vi "App - analyze RUS V6.vi"() -> ()   [LabVIEW 2021] (continued)
"Magn Field(T) "=0.0}, {"temperature"=14.72, "temperature str"="14.72000", "file path"=path "D:/Data/Ultrasound/LSCO/LSCO22__130814c/5_Cooling_2nd_try/September_2014/091714/14.72000K_500_2500_2.10000V_0.00000T_Sep17-2014__22-56-35_001_091714.bin", "last mod"=timestamp(3493853795 s since 1904-01-01), "file name str"="D:\\Data\\Ultrasound\\LSCO\\LSCO22__130814c\\5_Cooling_2nd_try\\September_2014\\091714\\14.72000K_500_2500_2.10000V_0.00000T_Sep17-2014__22-56-35_001_091714.bin", "mod time(min)"=58230896.583333336, "file format"=enum."binary", "power(V)"=2.1, "Magn Field(T) "=0.0}, {"temperature"=14.716, "temperature str"="14.71600", "file path"=path "D:/Data/Ultrasound/LSCO/LSCO22__130814c/5_Cooling_2nd_try/September_2014/091714/14.71600K_500_2500_2.10000V_0.00000T_Sep17-2014__22-57-54_001_091714.bin", "last mod"=timestamp(3493853874 s since 1904-01-01), "file name str"="D:\\Data\\Ultrasound\\LSCO\\LSCO22__130814c\\5_Cooling_2nd_try\\September_2014\\091714\\14.71600K_500_2500_2.10000V_0.00000T_Sep17-2014__22-57-54_001_091714.bin", "mod time(min)"=58230897.9, "file format"=enum."binary", "power(V)"=2.1, "Magn Field(T) "=0.0}, {"temperature"=14.713, "temperature str"="14.71300", "file path"=path "D:/Data/Ultrasound/LSCO/LSCO22__130814c/5_Cooling_2nd_try/September_2014/091714/14.71300K_500_2500_2.10000V_0.00000T_Sep17-2014__22-59-13_001_091714.bin", "last mod"=timestamp(3493853953 s since 1904-01-01), "file name str"="D:\\Data\\Ultrasound\\LSCO\\LSCO22__130814c\\5_Cooling_2nd_try\\September_2014\\091714\\14.71300K_500_2500_2.10000V_0.00000T_Sep17-2014__22-59-13_001_091714.bin", "mod time(min)"=58230899.21666667, "file format"=enum."binary", "power(V)"=2.1, "Magn Field(T) "=0.0}, {"temperature"=14.71, "temperature str"="14.71000", "file path"=path "D:/Data/Ultrasound/LSCO/LSCO22__130814c/5_Cooling_2nd_try/September_2014/091714/14.71000K_500_2500_2.10000V_0.00000T_Sep17-2014__23-00-33_001_091714.bin", "last mod"=timestamp(3493854033 s since 1904-01-01), "file name str"="D:\\Data\\Ultrasound\\LSCO\\LSCO22__130814c\\5_Cooling_2nd_try\\September_2014\\091714\\14.71000K_500_2500_2.10000V_0.00000T_Sep17-2014__23-00-33_001_091714.bin", "mod time(min)"=58230900.55, "file format"=enum."binary", "power(V)"=2.1, "Magn Field(T) "=0.0}, {"temperature"=14.704, "temperature str"="14.70400", "file path"=path "D:/Data/Ultrasound/LSCO/LSCO22__130814c/5_Cooling_2nd_try/September_2014/091714/14.70400K_500_2500_2.10000V_0.00000T_Sep17-2014__23-01-52_001_091714.bin", "last mod"=timestamp(3493854112 s since 1904-01-01), "file name str"="D:\\Data\\Ultrasound\\LSCO\\LSCO22__130814c\\5_Cooling_2nd_try\\September_2014\\091714\\14.70400K_500_2500_2.10000V_0.00000T_Sep17-2014__23-01-52_001_091714.bin", "mod time(min)"=58230901.86666667, "file format"=enum."binary", "power(V)"=2.1, "Magn Field(T) "=0.0}, {"temperature"=14.705, "temperature str"="14.70500", "file path"=path "D:/Data/Ultrasound/LSCO/LSCO22__130814c/5_Cooling_2nd_try/September_2014/091714/14.70500K_500_2500_2.10000V_0.00000T_Sep17-2014__23-03-11_001_091714.bin", "last mod"=timestamp(3493854191 s since 1904-01-01), "file name str"="D:\\Data\\Ultrasound\\LSCO\\LSCO22__130814c\\5_Cooling_2nd_try\\September_2014\\091714\\14.70500K_500_2500_2.10000V_0.00000T_Sep17-2014__23-03-11_001_091714.bin", "mod time(min)"=58230903.18333333, "file format"=enum."binary", "power(V)"=2.1, "Magn Field(T) "=0.0}, {"temperature"=14.703, "temperature str"="14.70300", "file path"=path "D:/Data/Ultrasound/LSCO/LSCO22__130814c/5_Cooling_2nd_try/September_2014/091714/14.70300K_500_2500_2.10000V_0.00000T_Sep17-2014__23-04-31_001_091714.bin", "last mod"=timestamp(3493854271 s since 1904-01-01), "file name str"="D:\\Data\\Ultrasound\\LSCO\\LSCO22__130814c\\5_Cooling_2nd_try\\September_2014\\091714\\14.70300K_500_2500_2.10000V_0.00000T_Sep17-2014__23-04-31_001_091714.bin", "mod time(min)"=58230904.516666666, "file format"=enum."binary", "power(V)"=2.1, "Magn Field(T) "=0.0}, {"temperature"=14.7, "temperature str"="14.70000", "file path"=path "D:/Data/Ultrasound/LSCO/LSCO22__130814c/5_Cooling_2nd_try/September_2014/091714/14.70000K_500_2500_2.10000V_0.00000T_Sep17-2014__23-05-50_001_091714.bin", "last mod"=timestamp(3493854350 s since 1904-01-01), "file name str"="D:\\Data\\Ultrasound\\LSCO\\LSCO22__130814c\\5_Cooling_2nd_try\\September_2014\\091714\\14.70000K_500_2500_2.10000V_0.00000T_Sep17-2014__23-05-50_001_091714.bin", "mod time(min)"=58230905.833333336, "file format"=enum."binary", "power(V)"=2.1, "Magn Field(T) "=0.0}, {"temperature"=14.697, "temperature str"="14.69700", "file path"=path "D:/Data/Ultrasound/LSCO/LSCO22__130814c/5_Cooling_2nd_try/September_2014/091714/14.69700K_500_2500_2.10000V_0.00000T_Sep17-2014__23-07-10_001_091714.bin", "last mod"=timestamp(3493854430 s since 1904-01-01), "file name str"="D:\\Data\\Ultrasound\\LSCO\\LSCO22__130814c\\5_Cooling_2nd_try\\September_2014\\091714\\14.69700K_500_2500_2.10000V_0.00000T_Sep17-2014__23-07-10_001_091714.bin", "mod time(min)"=58230907.166666664, "file format"=enum."binary", "power(V)"=2.1, "Magn Field(T) "=0.0}, {"temperature"=14.688, "temperature str"="14.68800", "file path"=path "D:/Data/Ultrasound/LSCO/LSCO22__130814c/5_Cooling_2nd_try/September_2014/091714/14.68800K_500_2500_2.10000V_0.00000T_Sep17-2014__23-08-29_001_091714.bin", "last mod"=timestamp(3493854509 s since 1904-01-01), "file name str"="D:\\Data\\Ultrasound\\LSCO\\LSCO22__130814c\\5_Cooling_2nd_try\\September_2014\\091714\\14.68800K_500_2500_2.10000V_0.00000T_Sep17-2014__23-08-29_001_091714.bin", "mod time(min)"=58230908.483333334, "file format"=enum."binary", "power(V)"=2.1, "Magn Field(T) "=0.0}, {"temperature"=14.695, "temperature str"="14.69500", "file path"=path "D:/Data/Ultrasound/LSCO/LSCO22__130814c/5_Cooling_2nd_try/September_2014/091714/14.69500K_500_2500_2.10000V_0.00000T_Sep17-2014__23-09-48_001_091714.bin", "last mod"=timestamp(3493854588 s since 1904-01-01), "file name str"="D:\\Data\\Ultrasound\\LSCO\\LSCO22__130814c\\5_Cooling_2nd_try\\September_2014\\091714\\14.69500K_500_2500_2.10000V_0.00000T_Sep17-2014__23-09-48_001_091714.bin", "mod time(min)"=58230909.8, "file format"=enum."binary", "power(V)"=2.1, "Magn Field(T) "=0.0}, {"temperature"=14.696, "temperature str"="14.69600", "file path"=path "D:/Data/Ultrasound/LSCO/LSCO22__130814c/5_Cooling_2nd_try/September_2014/091714/14.69600K_500_2500_2.10000V_0.00000T_Sep17-2014__23-11-08_001_091714.bin", "last mod"=timestamp(3493854668 s since 1904-01-01), "file name str"="D:\\Data\\Ultrasound\\LSCO\\LSCO22__130814c\\5_Cooling_2nd_try\\September_2014\\091714\\14.69600K_500_2500_2.10000V_0.00000T_Sep17-2014__23-11-08_001_091714.bin", "mod time(min)"=58230911.13333333, "file format"=enum."binary", "power(V)"=2.1, "Magn Field(T) "=0.0}, {"temperature"=14.691, "temperature str"="14.69100", "file path"=path "D:/Data/Ultrasound/LSCO/LSCO22__130814c/5_Cooling_2nd_try/September_2014/091714/14.69100K_500_2500_2.10000V_0.00000T_Sep17-2014__23-12-27_001_091714.bin", "last mod"=timestamp(3493854747 s since 1904-01-01), "file name str"="D:\\Data\\Ultrasound\\LSCO\\LSCO22__130814c\\5_Cooling_2nd_try\\September_2014\\091714\\14.69100K_500_2500_2.10000V_0.00000T_Sep17-2014__23-12-27_001_091714.bin", "mod time(min)"=58230912.45, "file format"=enum."binary", "power(V)"=2.1, "Magn Field(T) "=0.0}, {"temperature"=14.69, "temperature str"="14.69000", "file path"=path "D:/Data/Ultrasound/LSCO/LSCO22__130814c/5_Cooling_2nd_try/September_2014/091714/14.69000K_500_2500_2.10000V_0.00000T_Sep17-2014__23-13-46_001_091714.bin", "last mod"=timestamp(3493854826 s since 1904-01-01), "file name str"="D:\\Data\\Ultrasound\\LSCO\\LSCO22__130814c\\5_Cooling_2nd_try\\September_2014\\091714\\14.69000K_500_2500_2.10000V_0.00000T_Sep17-2014__23-13-46_001_091714.bin", "mod time(min)"=58230913.766666666, "file format"=enum."binary", "power(V)"=2.1, "Magn Field(T) "=0.0}, {"temperature"=14.69, "temperature str"="14.69000", "file path"=path "D:/Data/Ultrasound/LSCO/LSCO22__130814c/5_Cooling_2nd_try/September_2014/091714/14.69000K_500_2500_2.10000V_0.00000T_Sep17-2014__23-15-06_001_091714.bin", "last mod"=timestamp(3493854906 s since 1904-01-01), "file name str"="D:\\Data\\Ultrasound\\LSCO\\LSCO22__130814c\\5_Cooling_2nd_try\\September_2014\\091714\\14.69000K_500_2500_2.10000V_0.00000T_Sep17-2014__23-15-06_001_091714.bin", "mod time(min)"=58230915.1, "file format"=enum."binary", "power(V)"=2.1, "Magn Field(T) "=0.0}, {"temperature"=14.686, "temperature str"="14.68600", "file path"=path "D:/Data/Ultrasound/LSCO/LSCO22__130814c/5_Cooling_2nd_try/September_2014/091714/14.68600K_500_2500_2.10000V_0.00000T_Sep17-2014__23-16-25_001_091714.bin", "last mod"=timestamp(3493854985 s since 1904-01-01), "file name str"="D:\\Data\\Ultrasound\\LSCO\\LSCO22__130814c\\5_Cooling_2nd_try\\September_2014\\091714\\14.68600K_500_2500_2.10000V_0.00000T_Sep17-2014__23-16-25_001_091714.bin", "mod time(min)"=58230916.416666664, "file format"=enum."binary", "power(V)"=2.1, "Magn Field(T) "=0.0}, {"temperature"=14.682, "temperature str"="14.68200", "file path"=path "D:/Data/Ultrasound/LSCO/LSCO22__130814c/5_Cooling_2nd_try/September_2014/091714/14.68200K_500_2500_2.10000V_0.00000T_Sep17-2014__23-17-45_001_091714.bin", "last mod"=timestamp(3493855065 s since 1904-01-01), "file name str"="D:\\Data\\Ultrasound\\LSCO\\LSCO22__130814c\\5_Cooling_2nd_try\\September_2014\\091714\\14.68200K_500_2500_2.10000V_0.00000T_Sep17-2014__23-17-45_001_091714.bin", "mod time(min)"=58230917.75, "file format"=enum."binary", "power(V)"=2.1, "Magn Field(T) "=0.0}, {"temperature"=14.684, "temperature str"="14.68400", "file path"=path "D:/Data/Ultrasound/LSCO/LSCO22__130814c/5_Cooling_2nd_try/September_2014/091714/14.68400K_500_2500_2.10000V_0.00000T_Sep17-2014__23-19-04_001_091714.bin", "last mod"=timestamp(3493855144 s since 1904-01-01), "file name str"="D:\\Data\\Ultrasound\\LSCO\\LSCO22__130814c\\5_Cooling_2nd_try\\September_2014\\091714\\14.68400K_500_2500_2.10000V_0.00000T_Sep17-2014__23-19-04_001_091714.bin", "mod time(min)"=58230919.06666667, "file format"=enum."binary", "power(V)"=2.1, "Magn Field(T) "=0.0}, {"temperature"=14.679, "temperature str"="14.67900", "file path"=path "D:/Data/Ultrasound/LSCO/LSCO22__130814c/5_Cooling_2nd_try/September_2014/091714/14.67900K_500_2500_2.10000V_0.00000T_Sep17-2014__23-20-23_001_091714.bin", "last mod"=timestamp(3493855223 s since 1904-01-01), "file name str"="D:\\Data\\Ultrasound\\LSCO\\LSCO22__130814c\\5_Cooling_2nd_try\\September_2014\\091714\\14.67900K_500_2500_2.10000V_0.00000T_Sep17-2014__23-20-23_001_091714.bin", "mod time(min)"=58230920.38333333, "file format"=enum."binary", "power(V)"=2.1, "Magn Field(T) "=0.0}, {"temperature"=14.677, "temperature str"="14.67700", "file path"=path "D:/Data/Ultrasound/LSCO/LSCO22__130814c/5_Cooling_2nd_try/September_2014/091714/14.67700K_500_2500_2.10000V_0.00000T_Sep17-2014__23-21-43_001_091714.bin", "last mod"=timestamp(3493855303 s since 1904-01-01), "file name str"="D:\\Data\\Ultrasound\\LSCO\\LSCO22__130814c\\5_Cooling_2nd_try\\September_2014\\091714\\14.67700K_500_2500_2.10000V_0.00000T_Sep17-2014__23-21-43_001_091714.bin", "mod time(min)"=58230921.71666667, "file format"=enum."binary", "power(V)"=2.1, "Magn Field(T) "=0.0}, {"temperature"=14.676, "temperature str"="14.67600", "file path"=path "D:/Data/Ultrasound/LSCO/LSCO22__130814c/5_Cooling_2nd_try/September_2014/091714/14.67600K_500_2500_2.10000V_0.00000T_Sep17-2014__23-23-02_001_091714.bin", "last mod"=timestamp(3493855382 s since 1904-01-01), "file name str"="D:\\Data\\Ultrasound\\LSCO\\LSCO22__130814c\\5_Cooling_2nd_try\\September_2014\\091714\\14.67600K_500_2500_2.10000V_0.00000T_Sep17-2014__23-23-02_001_091714.bin", "mod time(min)"=58230923.03333333, "file format"=enum."binary", "power(V)"=2.1, "Magn Field(T) "=0.0}, {"temperature"=14.671, "temperature str"="14.67100", "file path"=path "D:/Data/Ultrasound/LSCO/LSCO22__130814c/5_Cooling_2nd_try/September_2014/091714/14.67100K_500_2500_2.10000V_0.00000T_Sep17-2014__23-24-22_001_091714.bin", "last mod"=timestamp(3493855462 s since 1904-01-01), "file name str"="D:\\Data\\Ultrasound\\LSCO\\LSCO22__130814c\\5_Cooling_2nd_try\\September_2014\\091714\\14.67100K_500_2500_2.10000V_0.00000T_Sep17-2014__23-24-22_001_091714.bin", "mod time(min)"=58230924.36666667, "file format"=enum."binary", "power(V)"=2.1, "Magn Field(T) "=0.0}, {"temperature"=14.665, "temperature str"="14.66500", "file path"=path "D:/Data/Ultrasound/LSCO/LSCO22__130814c/5_Cooling_2nd_try/September_2014/091714/14.66500K_500_2500_2.10000V_0.00000T_Sep17-2014__23-25-41_001_091714.bin", "last mod"=timestamp(3493855541 s since 1904-01-01), "file name str"="D:\\Data\\Ultrasound\\LSCO\\LSCO22__130814c\\5_Cooling_2nd_try\\September_2014\\091714\\14.66500K_500_2500_2.10000V_0.00000T_Sep17-2014__23-25-41_001_091714.bin", "mod time(min)"=58230925.68333333, "file format"=enum."binary", "power(V)"=2.1, "Magn Field(T) "=0.0}, {"temperature"=14.666, "temperature str"="14.66600", "file path"=path "D:/Data/Ultrasound/LSCO/LSCO22__130814c/5_Cooling_2nd_try/September_2014/091714/14.66600K_500_2500_2.10000V_0.00000T_Sep17-2014__23-27-00_001_091714.bin", "last mod"=timestamp(3493855620 s since 1904-01-01), "file name str"="D:\\Data\\Ultrasound\\LSCO\\LSCO22__130814c\\5_Cooling_2nd_try\\September_2014\\091714\\14.66600K_500_2500_2.10000V_0.00000T_Sep17-2014__23-27-00_001_091714.bin", "mod time(min)"=58230927.0, "file format"=enum."binary", "power(V)"=2.1, "Magn Field(T) "=0.0}, {"temperature"=14.661, "temperature str"="14.66100", "file path"=path "D:/Data/Ultrasound/LSCO/LSCO22__130814c/5_Cooling_2nd_try/September_2014/091714/14.66100K_500_2500_2.10000V_0.00000T_Sep17-2014__23-28-20_001_091714.bin", "last mod"=timestamp(3493855700 s since 1904-01-01), "file name str"="D:\\Data\\Ultrasound\\LSCO\\LSCO22__130814c\\5_Cooling_2nd_try\\September_2014\\091714\\14.66100K_500_2500_2.10000V_0.00000T_Sep17-2014__23-28-20_001_091714.bin", "mod time(min)"=58230928.333333336, "file format"=enum."binary", "power(V)"=2.1, "Magn Field(T) "=0.0}, {"temperature"=14.654, "temperature str"="14.65400", "file path"=path "D:/Data/Ultrasound/LSCO/LSCO22__130814c/5_Cooling_2nd_try/September_2014/091714/14.65400K_500_2500_2.10000V_0.00000T_Sep17-2014__23-29-39_001_091714.bin", "last mod"=timestamp(3493855779 s since 1904-01-01), "file name str"="D:\\Data\\Ultrasound\\LSCO\\LSCO22__130814c\\5_Cooling_2nd_try\\September_2014\\091714\\14.65400K_500_2500_2.10000V_0.00000T_Sep17-2014__23-29-39_001_091714.bin", "mod time(min)"=58230929.65, "file format"=enum."binary", "power(V)"=2.1, "Magn Field(T) "=0.0}, {"temperature"=14.654, "temperature str"="14.65400", "file path"=path "D:/Data/Ultrasound/LSCO/LSCO22__130814c/5_Cooling_2nd_try/September_2014/091714/14.65400K_500_2500_2.10000V_0.00000T_Sep17-2014__23-30-58_001_091714.bin", "last mod"=timestamp(3493855858 s since 1904-01-01), "file name str"="D:\\Data\\Ultrasound\\LSCO\\LSCO22__130814c\\5_Cooling_2nd_try\\September_2014\\091714\\14.65400K_500_2500_2.10000V_0.00000T_Sep17-2014__23-30-58_001_091714.bin", "mod time(min)"=58230930.96666667, "file format"=enum."binary", "power(V)"=2.1, "Magn Field(T) "=0.0}, {"temperature"=14.648, "temperature str"="14.64800", "file path"=path "D:/Data/Ultrasound/LSCO/LSCO22__130814c/5_Cooling_2nd_try/September_2014/091714/14.64800K_500_2500_2.10000V_0.00000T_Sep17-2014__23-32-18_001_091714.bin", "last mod"=timestamp(3493855938 s since 1904-01-01), "file name str"="D:\\Data\\Ultrasound\\LSCO\\LSCO22__130814c\\5_Cooling_2nd_try\\September_2014\\091714\\14.64800K_500_2500_2.10000V_0.00000T_Sep17-2014__23-32-18_001_091714.bin", "mod time(min)"=58230932.3, "file format"=enum."binary", "power(V)"=2.1, "Magn Field(T) "=0.0}, {"temperature"=14.653, "temperature str"="14.65300", "file path"=path "D:/Data/Ultrasound/LSCO/LSCO22__130814c/5_Cooling_2nd_try/September_2014/091714/14.65300K_500_2500_2.10000V_0.00000T_Sep17-2014__23-33-37_001_091714.bin", "last mod"=timestamp(3493856017 s since 1904-01-01), "file name str"="D:\\Data\\Ultrasound\\LSCO\\LSCO22__130814c\\5_Cooling_2nd_try\\September_2014\\091714\\14.65300K_500_2500_2.10000V_0.00000T_Sep17-2014__23-33-37_001_091714.bin", "mod time(min)"=58230933.61666667, "file format"=enum."binary", "power(V)"=2.1, "Magn Field(T) "=0.0}, {"temperature"=14.656, "temperature str"="14.65600", "file path"=path "D:/Data/Ultrasound/LSCO/LSCO22__130814c/5_Cooling_2nd_try/September_2014/091714/14.65600K_500_2500_2.10000V_0.00000T_Sep17-2014__23-34-57_001_091714.bin", "last mod"=timestamp(3493856097 s since 1904-01-01), "file name str"="D:\\Data\\Ultrasound\\LSCO\\LSCO22__130814c\\5_Cooling_2nd_try\\September_2014\\091714\\14.65600K_500_2500_2.10000V_0.00000T_Sep17-2014__23-34-57_001_091714.bin", "mod time(min)"=58230934.95, "file format"=enum."binary", "power(V)"=2.1, "Magn Field(T) "=0.0}, {"temperature"=14.654, "temperature str"="14.65400", "file path"=path "D:/Data/Ultrasound/LSCO/LSCO22__130814c/5_Cooling_2nd_try/September_2014/091714/14.65400K_500_2500_2.10000V_0.00000T_Sep17-2014__23-36-16_001_091714.bin", "last mod"=timestamp(3493856176 s since 1904-01-01), "file name str"="D:\\Data\\Ultrasound\\LSCO\\LSCO22__130814c\\5_Cooling_2nd_try\\September_2014\\091714\\14.65400K_500_2500_2.10000V_0.00000T_Sep17-2014__23-36-16_001_091714.bin", "mod time(min)"=58230936.266666666, "file format"=enum."binary", "power(V)"=2.1, "Magn Field(T) "=0.0}, {"temperature"=14.646, "temperature str"="14.64600", "file path"=path "D:/Data/Ultrasound/LSCO/LSCO22__130814c/5_Cooling_2nd_try/September_2014/091714/14.64600K_500_2500_2.10000V_0.00000T_Sep17-2014__23-37-35_001_091714.bin", "last mod"=timestamp(3493856255 s since 1904-01-01), "file name str"="D:\\Data\\Ultrasound\\LSCO\\LSCO22__130814c\\5_Cooling_2nd_try\\September_2014\\091714\\14.64600K_500_2500_2.10000V_0.00000T_Sep17-2014__23-37-35_001_091714.bin", "mod time(min)"=58230937.583333336, "file format"=enum."binary", "power(V)"=2.1, "Magn Field(T) "=0.0}, {"temperature"=14.643, "temperature str"="14.64300", "file path"=path "D:/Data/Ultrasound/LSCO/LSCO22__130814c/5_Cooling_2nd_try/September_2014/091714/14.64300K_500_2500_2.10000V_0.00000T_Sep17-2014__23-38-55_001_091714.bin", "last mod"=timestamp(3493856335 s since 1904-01-01), "file name str"="D:\\Data\\Ultrasound\\LSCO\\LSCO22__130814c\\5_Cooling_2nd_try\\September_2014\\091714\\14.64300K_500_2500_2.10000V_0.00000T_Sep17-2014__23-38-55_001_091714.bin", "mod time(min)"=58230938.916666664, "file format"=enum."binary", "power(V)"=2.1, "Magn Field(T) "=0.0}, {"temperature"=14.643, "temperature str"="14.64300", "file path"=path "D:/Data/Ultrasound/LSCO/LSCO22__130814c/5_Cooling_2nd_try/September_2014/091714/14.64300K_500_2500_2.10000V_0.00000T_Sep17-2014__23-40-14_001_091714.bin", "last mod"=timestamp(3493856414 s since 1904-01-01), "file name str"="D:\\Data\\Ultrasound\\LSCO\\LSCO22__130814c\\5_Cooling_2nd_try\\September_2014\\091714\\14.64300K_500_2500_2.10000V_0.00000T_Sep17-2014__23-40-14_001_091714.bin", "mod time(min)"=58230940.233333334, "file format"=enum."binary", "power(V)"=2.1, "Magn Field(T) "=0.0}, {"temperature"=14.638, "temperature str"="14.63800", "file path"=path "D:/Data/Ultrasound/LSCO/LSCO22__130814c/5_Cooling_2nd_try/September_2014/091714/14.63800K_500_2500_2.10000V_0.00000T_Sep17-2014__23-41-33_001_091714.bin", "last mod"=timestamp(3493856493 s since 1904-01-01), "file name str"="D:\\Data\\Ultrasound\\LSCO\\LSCO22__130814c\\5_Cooling_2nd_try\\September_2014\\091714\\14.63800K_500_2500_2.10000V_0.00000T_Sep17-2014__23-41-33_001_091714.bin", "mod time(min)"=58230941.55, "file format"=enum."binary", "power(V)"=2.1, "Magn Field(T) "=0.0}, {"temperature"=14.634, "temperature str"="14.63400", "file path"=path "D:/Data/Ultrasound/LSCO/LSCO22__130814c/5_Cooling_2nd_try/September_2014/091714/14.63400K_500_2500_2.10000V_0.00000T_Sep17-2014__23-42-53_001_091714.bin", "last mod"=timestamp(3493856573 s since 1904-01-01), "file name str"="D:\\Data\\Ultrasound\\LSCO\\LSCO22__130814c\\5_Cooling_2nd_try\\September_2014\\091714\\14.63400K_500_2500_2.10000V_0.00000T_Sep17-2014__23-42-53_001_091714.bin", "mod time(min)"=58230942.88333333, "file format"=enum."binary", "power(V)"=2.1, "Magn Field(T) "=0.0}, {"temperature"=14.63, "temperature str"="14.63000", "file path"=path "D:/Data/Ultrasound/LSCO/LSCO22__130814c/5_Cooling_2nd_try/September_2014/091714/14.63000K_500_2500_2.10000V_0.00000T_Sep17-2014__23-44-12_001_091714.bin", "last mod"=timestamp(3493856652 s since 1904-01-01), "file name str"="D:\\Data\\Ultrasound\\LSCO\\LSCO22__130814c\\5_Cooling_2nd_try\\September_2014\\091714\\14.63000K_500_2500_2.10000V_0.00000T_Sep17-2014__23-44-12_001_091714.bin", "mod time(min)"=58230944.2, "file format"=enum."binary", "power(V)"=2.1, "Magn Field(T) "=0.0}, {"temperature"=14.628, "temperature str"="14.62800", "file path"=path "D:/Data/Ultrasound/LSCO/LSCO22__130814c/5_Cooling_2nd_try/September_2014/091714/14.62800K_500_2500_2.10000V_0.00000T_Sep17-2014__23-45-32_001_091714.bin", "last mod"=timestamp(3493856732 s since 1904-01-01), "file name str"="D:\\Data\\Ultrasound\\LSCO\\LSCO22__130814c\\5_Cooling_2nd_try\\September_2014\\091714\\14.62800K_500_2500_2.10000V_0.00000T_Sep17-2014__23-45-32_001_091714.bin", "mod time(min)"=58230945.53333333, "file format"=enum."binary", "power(V)"=2.1, "Magn Field(T) "=0.0}, {"temperature"=14.626, "temperature str"="14.62600", "file path"=path "D:/Data/Ultrasound/LSCO/LSCO22__130814c/5_Cooling_2nd_try/September_2014/091714/14.62600K_500_2500_2.10000V_0.00000T_Sep17-2014__23-46-51_001_091714.bin", "last mod"=timestamp(3493856811 s since 1904-01-01), "file name str"="D:\\Data\\Ultrasound\\LSCO\\LSCO22__130814c\\5_Cooling_2nd_try\\September_2014\\091714\\14.62600K_500_2500_2.10000V_0.00000T_Sep17-2014__23-46-51_001_091714.bin", "mod time(min)"=58230946.85, "file format"=enum."binary", "power(V)"=2.1, "Magn Field(T) "=0.0}, {"temperature"=14.618, "temperature str"="14.61800", "file path"=path "D:/Data/Ultrasound/LSCO/LSCO22__130814c/5_Cooling_2nd_try/September_2014/091714/14.61800K_500_2500_2.10000V_0.00000T_Sep17-2014__23-48-10_001_091714.bin", "last mod"=timestamp(3493856890 s since 1904-01-01), "file name str"="D:\\Data\\Ultrasound\\LSCO\\LSCO22__130814c\\5_Cooling_2nd_try\\September_2014\\091714\\14.61800K_500_2500_2.10000V_0.00000T_Sep17-2014__23-48-10_001_091714.bin", "mod time(min)"=58230948.166666664, "file format"=enum."binary", "power(V)"=2.1, "Magn Field(T) "=0.0}, {"temperature"=14.618, "temperature str"="14.61800", "file path"=path "D:/Data/Ultrasound/LSCO/LSCO22__130814c/5_Cooling_2nd_try/September_2014/091714/14.61800K_500_2500_2.10000V_0.00000T_Sep17-2014__23-49-29_001_091714.bin", "last mod"=timestamp(3493856969 s since 1904-01-01), "file name str"="D:\\Data\\Ultrasound\\LSCO\\LSCO22__130814c\\5_Cooling_2nd_try\\September_2014\\091714\\14.61800K_500_2500_2.10000V_0.00000T_Sep17-2014__23-49-29_001_091714.bin", "mod time(min)"=58230949.483333334, "file format"=enum."binary", "power(V)"=2.1, "Magn Field(T) "=0.0}, {"temperature"=14.621, "temperature str"="14.62100", "file path"=path "D:/Data/Ultrasound/LSCO/LSCO22__130814c/5_Cooling_2nd_try/September_2014/091714/14.62100K_500_2500_2.10000V_0.00000T_Sep17-2014__23-50-49_001_091714.bin", "last mod"=timestamp(3493857049 s since 1904-01-01), "file name str"="D:\\Data\\Ultrasound\\LSCO\\LSCO22__130814c\\5_Cooling_2nd_try\\September_2014\\091714\\14.62100K_500_2500_2.10000V_0.00000T_Sep17-2014__23-50-49_001_091714.bin", "mod time(min)"=58230950.81666667, "file format"=enum."binary", "power(V)"=2.1, "Magn Field(T) "=0.0}, {"temperature"=14.616, "temperature str"="14.61600", "file path"=path "D:/Data/Ultrasound/LSCO/LSCO22__130814c/5_Cooling_2nd_try/September_2014/091714/14.61600K_500_2500_2.10000V_0.00000T_Sep17-2014__23-52-08_001_091714.bin", "last mod"=timestamp(3493857128 s since 1904-01-01), "file name str"="D:\\Data\\Ultrasound\\LSCO\\LSCO22__130814c\\5_Cooling_2nd_try\\September_2014\\091714\\14.61600K_500_2500_2.10000V_0.00000T_Sep17-2014__23-52-08_001_091714.bin", "mod time(min)"=58230952.13333333, "file format"=enum."binary", "power(V)"=2.1, "Magn Field(T) "=0.0}, {"temperature"=14.612, "temperature str"="14.61200", "file path"=path "D:/Data/Ultrasound/LSCO/LSCO22__130814c/5_Cooling_2nd_try/September_2014/091714/14.61200K_500_2500_2.10000V_0.00000T_Sep17-2014__23-53-27_001_091714.bin", "last mod"=timestamp(3493857207 s since 1904-01-01), "file name str"="D:\\Data\\Ultrasound\\LSCO\\LSCO22__130814c\\5_Cooling_2nd_try\\September_2014\\091714\\14.61200K_500_2500_2.10000V_0.00000T_Sep17-2014__23-53-27_001_091714.bin", "mod time(min)"=58230953.45, "file format"=enum."binary", "power(V)"=2.1, "Magn Field(T) "=0.0}, {"temperature"=14.606, "temperature str"="14.60600", "file path"=path "D:/Data/Ultrasound/LSCO/LSCO22__130814c/5_Cooling_2nd_try/September_2014/091714/14.60600K_500_2500_2.10000V_0.00000T_Sep17-2014__23-54-46_001_091714.bin", "last mod"=timestamp(3493857286 s since 1904-01-01), "file name str"="D:\\Data\\Ultrasound\\LSCO\\LSCO22__130814c\\5_Cooling_2nd_try\\September_2014\\091714\\14.60600K_500_2500_2.10000V_0.00000T_Sep17-2014__23-54-46_001_091714.bin", "mod time(min)"=58230954.766666666, "file format"=enum."binary", "power(V)"=2.1, "Magn Field(T) "=0.0}, {"temperature"=14.604, "temperature str"="14.60400", "file path"=path "D:/Data/Ultrasound/LSCO/LSCO22__130814c/5_Cooling_2nd_try/September_2014/091714/14.60400K_500_2500_2.10000V_0.00000T_Sep17-2014__23-56-06_001_091714.bin", "last mod"=timestamp(3493857366 s since 1904-01-01), "file name str"="D:\\Data\\Ultrasound\\LSCO\\LSCO22__130814c\\5_Cooling_2nd_try\\September_2014\\091714\\14.60400K_500_2500_2.10000V_0.00000T_Sep17-2014__23-56-06_001_091714.bin", "mod time(min)"=58230956.1, "file format"=enum."binary", "power(V)"=2.1, "Magn Field(T) "=0.0}, {"temperature"=14.604, "temperature str"="14.60400", "file path"=path "D:/Data/Ultrasound/LSCO/LSCO22__130814c/5_Cooling_2nd_try/September_2014/091714/14.60400K_500_2500_2.10000V_0.00000T_Sep17-2014__23-57-25_001_091714.bin", "last mod"=timestamp(3493857445 s since 1904-01-01), "file name str"="D:\\Data\\Ultrasound\\LSCO\\LSCO22__130814c\\5_Cooling_2nd_try\\September_2014\\091714\\14.60400K_500_2500_2.10000V_0.00000T_Sep17-2014__23-57-25_001_091714.bin", "mod time(min)"=58230957.416666664, "file format"=enum."binary", "power(V)"=2.1, "Magn Field(T) "=0.0}, {"temperature"=14.606, "temperature str"="14.60600", "file path"=path "D:/Data/Ultrasound/LSCO/LSCO22__130814c/5_Cooling_2nd_try/September_2014/091814/14.60600K_500_2500_2.10000V_0.00000T_Sep17-2014__23-58-44_001_091814.bin", "last mod"=timestamp(3493857524 s since 1904-01-01), "file name str"="D:\\Data\\Ultrasound\\LSCO\\LSCO22__130814c\\5_Cooling_2nd_try\\September_2014\\091814\\14.60600K_500_2500_2.10000V_0.00000T_Sep17-2014__23-58-44_001_091814.bin", "mod time(min)"=58230958.733333334, "file format"=enum."binary", "power(V)"=2.1, "Magn Field(T) "=0.0}, {"temperature"=14.605, "temperature str"="14.60500", "file path"=path "D:/Data/Ultrasound/LSCO/LSCO22__130814c/5_Cooling_2nd_try/September_2014/091814/14.60500K_500_2500_2.10000V_0.00000T_Sep18-2014__00-00-04_001_091814.bin", "last mod"=timestamp(3493857604 s since 1904-01-01), "file name str"="D:\\Data\\Ultrasound\\LSCO\\LSCO22__130814c\\5_Cooling_2nd_try\\September_2014\\091814\\14.60500K_500_2500_2.10000V_0.00000T_Sep18-2014__00-00-04_001_091814.bin", "mod time(min)"=58230960.06666667, "file format"=enum."binary", "power(V)"=2.1, "Magn Field(T) "=0.0}, {"temperature"=14.606, "temperature str"="14.60600", "file path"=path "D:/Data/Ultrasound/LSCO/LSCO22__130814c/5_Cooling_2nd_try/September_2014/091814/14.60600K_500_2500_2.10000V_0.00000T_Sep18-2014__00-01-23_001_091814.bin", "last mod"=timestamp(3493857683 s since 1904-01-01), "file name str"="D:\\Data\\Ultrasound\\LSCO\\LSCO22__130814c\\5_Cooling_2nd_try\\September_2014\\091814\\14.60600K_500_2500_2.10000V_0.00000T_Sep18-2014__00-01-23_001_091814.bin", "mod time(min)"=58230961.38333333, "file format"=enum."binary", "power(V)"=2.1, "Magn Field(T) "=0.0}, {"temperature"=14.603, "temperature str"="14.60300", "file path"=path "D:/Data/Ultrasound/LSCO/LSCO22__130814c/5_Cooling_2nd_try/September_2014/091814/14.60300K_500_2500_2.10000V_0.00000T_Sep18-2014__00-02-42_001_091814.bin", "last mod"=timestamp(3493857762 s since 1904-01-01), "file name str"="D:\\Data\\Ultrasound\\LSCO\\LSCO22__130814c\\5_Cooling_2nd_try\\September_2014\\091814\\14.60300K_500_2500_2.10000V_0.00000T_Sep18-2014__00-02-42_001_091814.bin", "mod time(min)"=58230962.7, "file format"=enum."binary", "power(V)"=2.1, "Magn Field(T) "=0.0}, {"temperature"=14.6, "temperature str"="14.60000", "file path"=path "D:/Data/Ultrasound/LSCO/LSCO22__130814c/5_Cooling_2nd_try/September_2014/091814/14.60000K_500_2500_2.10000V_0.00000T_Sep18-2014__00-04-02_001_091814.bin", "last mod"=timestamp(3493857842 s since 1904-01-01), "file name str"="D:\\Data\\Ultrasound\\LSCO\\LSCO22__130814c\\5_Cooling_2nd_try\\September_2014\\091814\\14.60000K_500_2500_2.10000V_0.00000T_Sep18-2014__00-04-02_001_091814.bin", "mod time(min)"=58230964.03333333, "file format"=enum."binary", "power(V)"=2.1, "Magn Field(T) "=0.0}, {"temperature"=14.601, "temperature str"="14.60100", "file path"=path "D:/Data/Ultrasound/LSCO/LSCO22__130814c/5_Cooling_2nd_try/September_2014/091814/14.60100K_500_2500_2.10000V_0.00000T_Sep18-2014__00-05-21_001_091814.bin", "last mod"=timestamp(3493857921 s since 1904-01-01), "file name str"="D:\\Data\\Ultrasound\\LSCO\\LSCO22__130814c\\5_Cooling_2nd_try\\September_2014\\091814\\14.60100K_500_2500_2.10000V_0.00000T_Sep18-2014__00-05-21_001_091814.bin", "mod time(min)"=58230965.35, "file format"=enum."binary", "power(V)"=2.1, "Magn Field(T) "=0.0}, {"temperature"=14.595, "temperature str"="14.59500", "file path"=path "D:/Data/Ultrasound/LSCO/LSCO22__130814c/5_Cooling_2nd_try/September_2014/091814/14.59500K_500_2500_2.10000V_0.00000T_Sep18-2014__00-06-40_001_091814.bin", "last mod"=timestamp(3493858000 s since 1904-01-01), "file name str"="D:\\Data\\Ultrasound\\LSCO\\LSCO22__130814c\\5_Cooling_2nd_try\\September_2014\\091814\\14.59500K_500_2500_2.10000V_0.00000T_Sep18-2014__00-06-40_001_091814.bin", "mod time(min)"=58230966.666666664, "file format"=enum."binary", "power(V)"=2.1, "Magn Field(T) "=0.0}, {"temperature"=14.592, "temperature str"="14.59200", "file path"=path "D:/Data/Ultrasound/LSCO/LSCO22__130814c/5_Cooling_2nd_try/September_2014/091814/14.59200K_500_2500_2.10000V_0.00000T_Sep18-2014__00-08-00_001_091814.bin", "last mod"=timestamp(3493858080 s since 1904-01-01), "file name str"="D:\\Data\\Ultrasound\\LSCO\\LSCO22__130814c\\5_Cooling_2nd_try\\September_2014\\091814\\14.59200K_500_2500_2.10000V_0.00000T_Sep18-2014__00-08-00_001_091814.bin", "mod time(min)"=58230968.0, "file format"=enum."binary", "power(V)"=2.1, "Magn Field(T) "=0.0}, {"temperature"=14.59, "temperature str"="14.59000", "file path"=path "D:/Data/Ultrasound/LSCO/LSCO22__130814c/5_Cooling_2nd_try/September_2014/091814/14.59000K_500_2500_2.10000V_0.00000T_Sep18-2014__00-09-19_001_091814.bin", "last mod"=timestamp(3493858159 s since 1904-01-01), "file name str"="D:\\Data\\Ultrasound\\LSCO\\LSCO22__130814c\\5_Cooling_2nd_try\\September_2014\\091814\\14.59000K_500_2500_2.10000V_0.00000T_Sep18-2014__00-09-19_001_091814.bin", "mod time(min)"=58230969.31666667, "file format"=enum."binary", "power(V)"=2.1, "Magn Field(T) "=0.0}, {"temperature"=14.588, "temperature str"="14.58800", "file path"=path "D:/Data/Ultrasound/LSCO/LSCO22__130814c/5_Cooling_2nd_try/September_2014/091814/14.58800K_500_2500_2.10000V_0.00000T_Sep18-2014__00-10-38_001_091814.bin", "last mod"=timestamp(3493858238 s since 1904-01-01), "file name str"="D:\\Data\\Ultrasound\\LSCO\\LSCO22__130814c\\5_Cooling_2nd_try\\September_2014\\091814\\14.58800K_500_2500_2.10000V_0.00000T_Sep18-2014__00-10-38_001_091814.bin", "mod time(min)"=58230970.63333333, "file format"=enum."binary", "power(V)"=2.1, "Magn Field(T) "=0.0}, {"temperature"=14.586, "temperature str"="14.58600", "file path"=path "D:/Data/Ultrasound/LSCO/LSCO22__130814c/5_Cooling_2nd_try/September_2014/091814/14.58600K_500_2500_2.10000V_0.00000T_Sep18-2014__00-11-58_001_091814.bin", "last mod"=timestamp(3493858318 s since 1904-01-01), "file name str"="D:\\Data\\Ultrasound\\LSCO\\LSCO22__130814c\\5_Cooling_2nd_try\\September_2014\\091814\\14.58600K_500_2500_2.10000V_0.00000T_Sep18-2014__00-11-58_001_091814.bin", "mod time(min)"=58230971.96666667, "file format"=enum."binary", "power(V)"=2.1, "Magn Field(T) "=0.0}, {"temperature"=14.583, "temperature str"="14.58300", "file path"=path "D:/Data/Ultrasound/LSCO/LSCO22__130814c/5_Cooling_2nd_try/September_2014/091814/14.58300K_500_2500_2.10000V_0.00000T_Sep18-2014__00-13-17_001_091814.bin", "last mod"=timestamp(3493858397 s since 1904-01-01), "file name str"="D:\\Data\\Ultrasound\\LSCO\\LSCO22__130814c\\5_Cooling_2nd_try\\September_2014\\091814\\14.58300K_500_2500_2.10000V_0.00000T_Sep18-2014__00-13-17_001_091814.bin", "mod time(min)"=58230973.28333333, "file format"=enum."binary", "power(V)"=2.1, "Magn Field(T) "=0.0}, {"temperature"=14.577, "temperature str"="14.57700", "file path"=path "D:/Data/Ultrasound/LSCO/LSCO22__130814c/5_Cooling_2nd_try/September_2014/091814/14.57700K_500_2500_2.10000V_0.00000T_Sep18-2014__00-14-37_001_091814.bin", "last mod"=timestamp(3493858477 s since 1904-01-01), "file name str"="D:\\Data\\Ultrasound\\LSCO\\LSCO22__130814c\\5_Cooling_2nd_try\\September_2014\\091814\\14.57700K_500_2500_2.10000V_0.00000T_Sep18-2014__00-14-37_001_091814.bin", "mod time(min)"=58230974.61666667, "file format"=enum."binary", "power(V)"=2.1, "Magn Field(T) "=0.0}, {"temperature"=14.575, "temperature str"="14.57500", "file path"=path "D:/Data/Ultrasound/LSCO/LSCO22__130814c/5_Cooling_2nd_try/September_2014/091814/14.57500K_500_2500_2.10000V_0.00000T_Sep18-2014__00-15-56_001_091814.bin", "last mod"=timestamp(3493858556 s since 1904-01-01), "file name str"="D:\\Data\\Ultrasound\\LSCO\\LSCO22__130814c\\5_Cooling_2nd_try\\September_2014\\091814\\14.57500K_500_2500_2.10000V_0.00000T_Sep18-2014__00-15-56_001_091814.bin", "mod time(min)"=58230975.93333333, "file format"=enum."binary", "power(V)"=2.1, "Magn Field(T) "=0.0}, {"temperature"=14.575, "temperature str"="14.57500", "file path"=path "D:/Data/Ultrasound/LSCO/LSCO22__130814c/5_Cooling_2nd_try/September_2014/091814/14.57500K_500_2500_2.10000V_0.00000T_Sep18-2014__00-17-15_001_091814.bin", "last mod"=timestamp(3493858635 s since 1904-01-01), "file name str"="D:\\Data\\Ultrasound\\LSCO\\LSCO22__130814c\\5_Cooling_2nd_try\\September_2014\\091814\\14.57500K_500_2500_2.10000V_0.00000T_Sep18-2014__00-17-15_001_091814.bin", "mod time(min)"=58230977.25, "file format"=enum."binary", "power(V)"=2.1, "Magn Field(T) "=0.0}, {"temperature"=14.572, "temperature str"="14.57200", "file path"=path "D:/Data/Ultrasound/LSCO/LSCO22__130814c/5_Cooling_2nd_try/September_2014/091814/14.57200K_500_2500_2.10000V_0.00000T_Sep18-2014__00-18-35_001_091814.bin", "last mod"=timestamp(3493858715 s since 1904-01-01), "file name str"="D:\\Data\\Ultrasound\\LSCO\\LSCO22__130814c\\5_Cooling_2nd_try\\September_2014\\091814\\14.57200K_500_2500_2.10000V_0.00000T_Sep18-2014__00-18-35_001_091814.bin", "mod time(min)"=58230978.583333336, "file format"=enum."binary", "power(V)"=2.1, "Magn Field(T) "=0.0}, {"temperature"=14.574, "temperature str"="14.57400", "file path"=path "D:/Data/Ultrasound/LSCO/LSCO22__130814c/5_Cooling_2nd_try/September_2014/091814/14.57400K_500_2500_2.10000V_0.00000T_Sep18-2014__00-19-54_001_091814.bin", "last mod"=timestamp(3493858794 s since 1904-01-01), "file name str"="D:\\Data\\Ultrasound\\LSCO\\LSCO22__130814c\\5_Cooling_2nd_try\\September_2014\\091814\\14.57400K_500_2500_2.10000V_0.00000T_Sep18-2014__00-19-54_001_091814.bin", "mod time(min)"=58230979.9, "file format"=enum."binary", "power(V)"=2.1, "Magn Field(T) "=0.0}, {"temperature"=14.57, "temperature str"="14.57000", "file path"=path "D:/Data/Ultrasound/LSCO/LSCO22__130814c/5_Cooling_2nd_try/September_2014/091814/14.57000K_500_2500_2.10000V_0.00000T_Sep18-2014__00-21-13_001_091814.bin", "last mod"=timestamp(3493858873 s since 1904-01-01), "file name str"="D:\\Data\\Ultrasound\\LSCO\\LSCO22__130814c\\5_Cooling_2nd_try\\September_2014\\091814\\14.57000K_500_2500_2.10000V_0.00000T_Sep18-2014__00-21-13_001_091814.bin", "mod time(min)"=58230981.21666667, "file format"=enum."binary", "power(V)"=2.1, "Magn Field(T) "=0.0}, {"temperature"=14.574, "temperature str"="14.57400", "file path"=path "D:/Data/Ultrasound/LSCO/LSCO22__130814c/5_Cooling_2nd_try/September_2014/091814/14.57400K_500_2500_2.10000V_0.00000T_Sep18-2014__00-22-33_001_091814.bin", "last mod"=timestamp(3493858953 s since 1904-01-01), "file name str"="D:\\Data\\Ultrasound\\LSCO\\LSCO22__130814c\\5_Cooling_2nd_try\\September_2014\\091814\\14.57400K_500_2500_2.10000V_0.00000T_Sep18-2014__00-22-33_001_091814.bin", "mod time(min)"=58230982.55, "file format"=enum."binary", "power(V)"=2.1, "Magn Field(T) "=0.0}, {"temperature"=14.576, "temperature str"="14.57600", "file path"=path "D:/Data/Ultrasound/LSCO/LSCO22__130814c/5_Cooling_2nd_try/September_2014/091814/14.57600K_500_2500_2.10000V_0.00000T_Sep18-2014__00-23-52_001_091814.bin", "last mod"=timestamp(3493859032 s since 1904-01-01), "file name str"="D:\\Data\\Ultrasound\\LSCO\\LSCO22__130814c\\5_Cooling_2nd_try\\September_2014\\091814\\14.57600K_500_2500_2.10000V_0.00000T_Sep18-2014__00-23-52_001_091814.bin", "mod time(min)"=58230983.86666667, "file format"=enum."binary", "power(V)"=2.1, "Magn Field(T) "=0.0}, {"temperature"=14.575, "temperature str"="14.57500", "file path"=path "D:/Data/Ultrasound/LSCO/LSCO22__130814c/5_Cooling_2nd_try/September_2014/091814/14.57500K_500_2500_2.10000V_0.00000T_Sep18-2014__00-25-12_001_091814.bin", "last mod"=timestamp(3493859112 s since 1904-01-01), "file name str"="D:\\Data\\Ultrasound\\LSCO\\LSCO22__130814c\\5_Cooling_2nd_try\\September_2014\\091814\\14.57500K_500_2500_2.10000V_0.00000T_Sep18-2014__00-25-12_001_091814.bin", "mod time(min)"=58230985.2, "file format"=enum."binary", "power(V)"=2.1, "Magn Field(T) "=0.0}, {"temperature"=14.567, "temperature str"="14.56700", "file path"=path "D:/Data/Ultrasound/LSCO/LSCO22__130814c/5_Cooling_2nd_try/September_2014/091814/14.56700K_500_2500_2.10000V_0.00000T_Sep18-2014__00-26-31_001_091814.bin", "last mod"=timestamp(3493859191 s since 1904-01-01), "file name str"="D:\\Data\\Ultrasound\\LSCO\\LSCO22__130814c\\5_Cooling_2nd_try\\September_2014\\091814\\14.56700K_500_2500_2.10000V_0.00000T_Sep18-2014__00-26-31_001_091814.bin", "mod time(min)"=58230986.516666666, "file format"=enum."binary", "power(V)"=2.1, "Magn Field(T) "=0.0}, {"temperature"=14.572, "temperature str"="14.57200", "file path"=path "D:/Data/Ultrasound/LSCO/LSCO22__130814c/5_Cooling_2nd_try/September_2014/091814/14.57200K_500_2500_2.10000V_0.00000T_Sep18-2014__00-27-50_001_091814.bin", "last mod"=timestamp(3493859270 s since 1904-01-01), "file name str"="D:\\Data\\Ultrasound\\LSCO\\LSCO22__130814c\\5_Cooling_2nd_try\\September_2014\\091814\\14.57200K_500_2500_2.10000V_0.00000T_Sep18-2014__00-27-50_001_091814.bin", "mod time(min)"=58230987.833333336, "file format"=enum."binary", "power(V)"=2.1, "Magn Field(T) "=0.0}, {"temperature"=14.571, "temperature str"="14.57100", "file path"=path "D:/Data/Ultrasound/LSCO/LSCO22__130814c/5_Cooling_2nd_try/September_2014/091814/14.57100K_500_2500_2.10000V_0.00000T_Sep18-2014__00-29-10_001_091814.bin", "last mod"=timestamp(3493859350 s since 1904-01-01), "file name str"="D:\\Data\\Ultrasound\\LSCO\\LSCO22__130814c\\5_Cooling_2nd_try\\September_2014\\091814\\14.57100K_500_2500_2.10000V_0.00000T_Sep18-2014__00-29-10_001_091814.bin", "mod time(min)"=58230989.166666664, "file format"=enum."binary", "power(V)"=2.1, "Magn Field(T) "=0.0}, {"temperature"=14.568, "temperature str"="14.56800", "file path"=path "D:/Data/Ultrasound/LSCO/LSCO22__130814c/5_Cooling_2nd_try/September_2014/091814/14.56800K_500_2500_2.10000V_0.00000T_Sep18-2014__00-30-29_001_091814.bin", "last mod"=timestamp(3493859429 s since 1904-01-01), 
